vi "Index Count_In Time Range.vi"(5 "Open(t) Closed(f)":bool, 7 "Dt":dbl, 10 "Tf":timestamp, 11 "T0":timestamp) -> (3 "Numeric":i32)   [LabVIEW 2020]
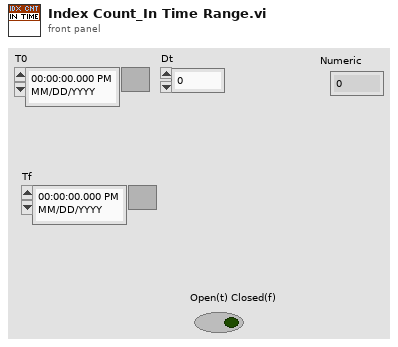
[diagram p1: front panel]
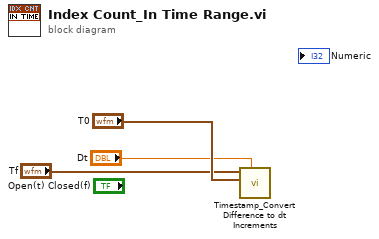
[diagram p0: block diagram]
diagram:
  n1 = call "Timestamp_Convert Difference to dt Increments.vi"("Dt"="Dt", "Start Time"="T0", "End Time"="Tf") -> ()  [unwired: 6 in, 3 out]
